vi "Do.vi"(8 "error in (no error)":errorcluster, 10 "Actor in":refnum<class "Actor.lvclass">, 11 "Configure FM Enabled [FM] Msg":refnum<class "Configure FM Enabled [FM] Msg.lvclass">) -> (0 "error out":errorcluster, 2 "Actor out":refnum<class "Actor.lvclass">)   [LabVIEW 2016, in "CS++Fgen.lvlib" / "Configure FM Enabled [FM] Msg.lvclass"]
doc: "This VI delivers the message to the actor by calling the appropriate method(s) on the actor."
uses:
  Configure FM Enabled [FM] Msg.lvclass
  <vilib>/ActorFramework/Actor/Actor.lvclass
  C:/User/Brand/LVP/CSPP-Dev/Packages/CSPP_Core/Actors/CS++PVMonitor Messages/CS++PVUpdate Msg/CS++PVUpdate Msg.lvclass
  CS++Fgen/CS++Fgen.lvclass
  C:/Program Files (x86)/National Instruments/LabVIEW 2016/vi.lib/ActorFramework/Actor/Actor.lvclass
  CSPP_Core/Actors/CS++PVMonitor Messages/CS++PVUpdate Msg/CS++PVUpdate Msg.lvclass/CS++PVUpdate Msg.ctl
  CSPP_Core/Classes/CS++ProcessVariables/ProcessVariable/PV.lvclass/PV.ctl
  Configure FM Enabled [FM] Msg.lvclass/Configure FM Enabled [FM] Msg.ctl
  CSPP_Core/Classes/CS++ProcessVariables/ProcessVariable/PV.lvclass
  CSPP_Core/Actors/CS++PVMonitor Messages/CS++PVUpdate Msg/CS++PVUpdate Msg.lvclass
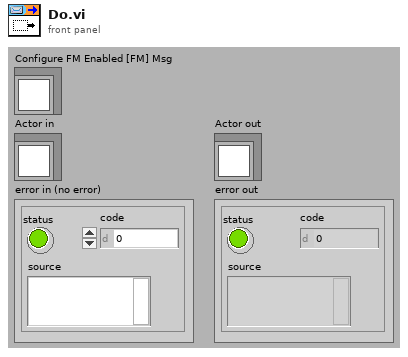
[diagram p1: front panel]
types:
  T1 = cluster{"Channel Name (\"\")":string, "FM enabled (True)":bool}
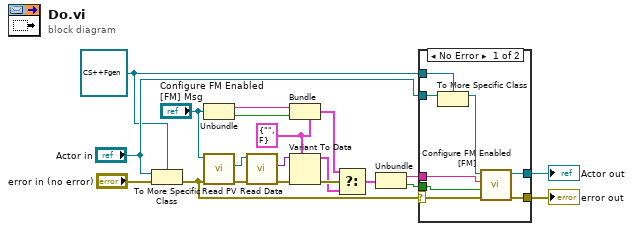
[diagram p0: block diagram]
diagram:
  w12 = T1 {"Channel Name (\"\")"="", "FM enabled (True)"=FALSE} ("Type")
  w16 = refnum<class "CS++Fgen.lvclass"> refnum ("Actor in")
  n1 = To More Specific Class(target class=w16, reference="Actor in", error in="error in (no error)") -> (error out=w5:errorcluster)  [unwired: 1 out]
  n2 = Unbundle ("Pre-Unbundler")("Configure FM Enabled [FM] Msg") -> (w3:string, w2:bool)
  n3 = call "Read PV.vi"("error in (no error)"=w5, "CS++PVUpdate Msg in"="Configure FM Enabled [FM] Msg") -> ("error out"=w15:errorcluster, "PV"=w11:refnum<class "PV.lvclass">)  [unwired: 7 in, 1 out]
  n4 = call "Read Data.vi"("error in (no error)"=w15, "PV in"=w11) -> ("error out"=w9:errorcluster, "Data"=w10:variant)  [unwired: 7 in, 1 out]
  n5 = Bundle ("Pre-Bundler")(cluster=w12, "Channel Name (\"\")"=w3, "FM enabled (True)"=w2) -> (w13:T1)
  n6 = Variant To Data(error in=w9, type=w12, Variant=w10) -> (data=w7:T1, error out=w14:errorcluster)
  n7 = Select ("MainSelect")(t=w13, s=w14, f=w7) -> (s? t:f=w8:T1)
  n8 = Unbundle ("Main-Unbundler")(w8) -> ("Channel Name (\"\")"=w4:string, "FM enabled (True)"=w1:bool)
  n9 = case shown="No Error" w5 {
    selector: w5 -> [w26 w30]
    tunnel: [w28 w30] -> w19
    tunnel: [w27 w29] -> w18
    tunnel: "Actor in" -> [w25 w29]
    tunnel: w16 -> [w24 _]
    tunnel: w4 -> [w22 _]
    tunnel: w1 -> [w21 _]
    frame No Error {
      n10 = To More Specific Class(target class=w24, reference=w25) -> (specific class reference=w23:refnum<class "CS++Fgen.lvclass">)  [unwired: 1 in, 1 out]
      n11 = call "Configure FM Enabled [FM].vi"("error in (no error)"=w26, "FM enabled (True)"=w21, "Channel Name (\"\")"=w22, "CS++Fgen in"=w23) -> ("error out"=w28:errorcluster, "CS++Fgen out"=w27:refnum<class "CS++Fgen.lvclass">)  [unwired: 6 in]
    }
    frame Error {
    }
  }
  "error out" <- w19
  "Actor out" <- w18
